vi "21-RollScoreDistributions.vi"(10 "Rolls Per Turn":i32, 11 "Dice Positions":i32) -> (2 "DU":u64[](array[numeric]), 3 "D":u64[](array[numeric]))   [LabVIEW 2019, in "21.lvlib"]
uses:
  21.lvlib
  <vilib>/Analysis/NI_AALBase.lvlib
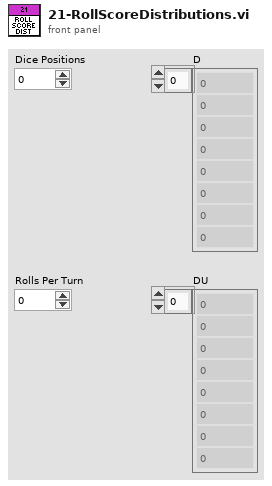
[diagram p1: front panel]
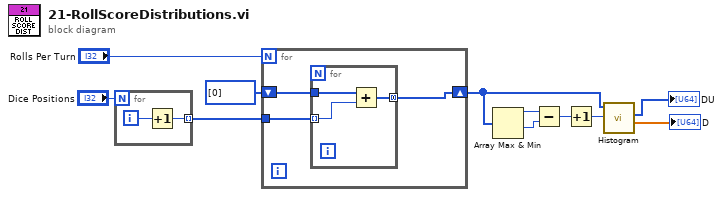
[diagram p0: block diagram]
diagram:
  n1 = for {
    N: "Dice Positions" -> [_]
    tunnel: [w12] -> w9 mode=indexing
    i -> [w13]
    n2 = Increment(x=w13) -> (x+1=w12:i32)
  }
  n3 = for {
    N: "Rolls Per Turn" -> [_]
    tunnel: w9 -> [w16]
    shift-right: [w15] -> w7
    shift-left: i32[] [0] -> [w14]
    n4 = for {
      tunnel: w16 -> [w19] mode=indexing
      tunnel: [w18] -> w15 mode=concatenating
      tunnel: w14 -> [w17]
      n5 = Add(x=w17, y=w19) -> (x+y=w18:i32[])
    }
  }
  n6 = Array Max & Min(array=w7) -> (max value=w5:i32, min value=w6:i32)  [unwired: 2 out]
  n7 = Subtract(x=w5, y=w6) -> (x-y=w4:i32)
  n8 = Increment(x=w4) -> (x+1=w1:i32)
  n9 = call <vilib>:"Histogram.vi"("intervals"=w1, "X"=w7) -> ("X Values"=→"D":dbl[], "Histogram: h(x)"=→"DU":i32[])  [unwired: 6 in, 2 out]
